vi "Construct.vi"(8 "error in (no error)":errorcluster, 11 "parameters":T1) -> (0 "error out":errorcluster, 3 "NI-XNET CAN Reader Execution Unit":refnum<class "NI-XNET CAN Reader Execution Unit.lvclass">)   [LabVIEW 2020, in "Communication Bus Template Engine.lvlib" / "Implementation.lvlib" / "NI-XNET CAN Reader Execution Unit.lvclass"]
uses:
  NI-XNET CAN Reader Execution Unit.lvclass
  Parameters.ctl
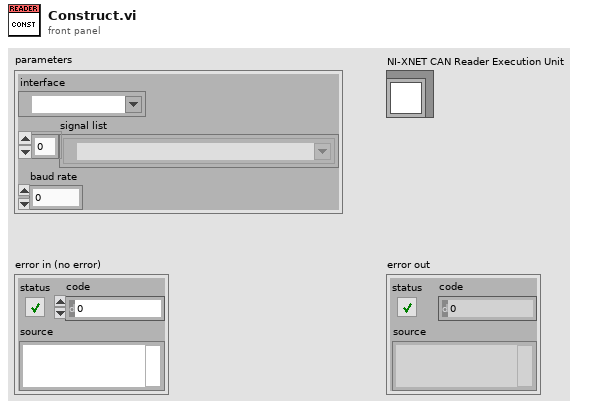
[diagram p1: front panel]
types:
  T1 = typedef "Communication Bus Template Engine.lvlib/Implementation.lvlib/NI-XNET CAN Reader Execution Unit.lvclass/Parameters.ctl" = cluster{"interface":refnum<k21>, "signal list":refnum<k21>[], "baud rate":u64}
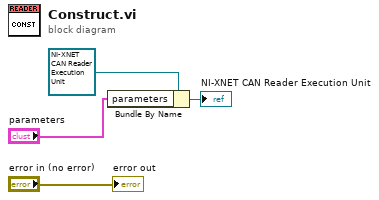
[diagram p0: block diagram]
diagram:
  n1 = Bundle By Name(cluster=refnum<class "NI-XNET CAN Reader Execution Unit.lvclass"> refnum ("Communication Bus Template Interfaces:Implementation.lvlib:NI-XNET CAN Reader Execution Unit.lvclass"), "parameters"="parameters") -> (→"NI-XNET CAN Reader Execution Unit":refnum<class "NI-XNET CAN Reader Execution Unit.lvclass">)
  "error out" <- "error in (no error)"
